vi "Read Source.vi"(11 "Move in":refnum<class "Move.lvclass">) -> (2 "Square":T1={"File"=enum."d", "Rank"=enum."4"}, 3 "Move out":refnum<class "Move.lvclass">)   [LabVIEW 2016, in "Chesslib.lvlib" / "Move.lvclass"]
uses:
  Move.lvclass
  typedef/Square.ctl
  typedef/File.ctl
  typedef/Rank.ctl
  Move.lvclass/Move.ctl
  Chesslib.lvlib
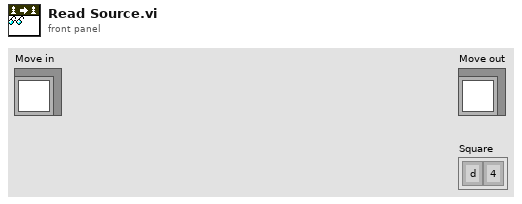
[diagram p1: front panel]
types:
  T1 = typedef "Chesslib.lvlib/Square.ctl" = cluster{"File":T2, "Rank":T3}
  T2 = typedef "Chesslib.lvlib/File.ctl" = enum8{"a", "b", "c", "d", "e", "f", "g", "h"}
  T3 = typedef "Chesslib.lvlib/Rank.ctl" = enum8{"1", "2", "3", "4", "5", "6", "7", "8"}
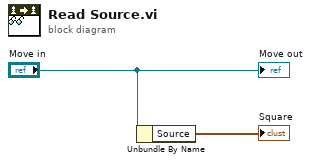
[diagram p0: block diagram]
diagram:
  n1 = Unbundle By Name("Move in") -> ("Source"=→"Square":T1)
  "Move out" <- "Move in"
